vi "诊断标定3 - 副本.vi"(8 "CAN端口":u16(ring), 9 "设备索引号":u16(ring), 10 "CAN卡类型":u32(ring)=21) -> ()   [LabVIEW 2013] (continued)
                n2793 = local read "CAN卡类型"() -> (w3541:u32)
                n2794 = local read "CAN端口"() -> (w3539:u16)
                n2795 = call "标定授权发送.vi"("CAN卡类型"=w3541, "解锁类型"=enum16{"读取", "写", "下载"}."写", "设备索引号"=w3540, "CAN端口"=w3539, "是否连接"=TRUE, "板选择"=0, "FUNC"=w3543) -> ("发送成功"=w3546:bool)  [unwired: 8 out]
              }
              frame Enabled {
              }
            }
            n2796 = case shown="真" w3533 {
              tunnel: w3537 -> [w3551 w3556]
              tunnel: w3536 -> [w3550 w3555]
              tunnel: [w3551 w3553] -> w3535
              tunnel: [w3550 w3552] -> w3534
              frame False {
              }
              frame True {
                n2797 = Enqueue Element(queue=w3556, element="读取故障状态" ("元素"), error in (no error)=w3555) -> (queue out=w3553:refnum<queue>, error out=w3552:errorcluster)  [unwired: 2 out]
              }
            }
            n2798 = local write "电池故障"(string[][] []) -> ()
            n2799 = global write "EV05全局变量1.vi" "流控帧 2"(TRUE ("流控帧")) -> ()
            n2800 = local write "写?"(FALSE ("写?")) -> ()
            n2801 = local write "控制1"(TRUE ("控制1")) -> ()
            n2802 = local write "消除"(TRUE ("消除")) -> ()
            n2803 = local write "清BUFF"(FALSE ("清BUFF")) -> ()
            n2804 = global write "EV05全局变量1.vi" "流控帧"(FALSE ("流控帧")) -> ()
            n2805 = call <vilib>:"Set Busy.vi"("disable click? (T)"=FALSE) -> ()  [unwired: 3 in, 8 out]
          }
        }
      }
      event "项目软本读取": Value Change {
        n2806 = event-data() -> ("NewVal"=w3561:bool)  [unwired: 5 out]
        n2807 = case shown="真" w3561 {
          tunnel: w3560 -> [w3563 w3570]
          tunnel: w3559 -> [w3562 w3569]
          tunnel: [w3563 w3568] -> w3558
          tunnel: [w3562 w3567] -> w3557
          frame False {
          }
          frame True {
            n2808 = global read "EV05全局变量1.vi" "授权功能"() -> (w3565:bool)
            n2809 = case shown="假" w3565 {
              tunnel: [TRUE ("发送成功") w3589] -> w3566
              frame False {
              }
              frame True {
                n2810 = local read "设备索引号"() -> (w3584:u16)
                n2811 = local read "CAN卡类型"() -> (w3585:u32)
                n2812 = local read "CAN端口"() -> (w3583:u16)
                n2813 = call "标定授权发送.vi"("CAN卡类型"=w3585, "解锁类型"=enum16{"读取", "写", "下载"}."读取", "设备索引号"=w3584, "CAN端口"=w3583, "是否连接"=TRUE, "板选择"=0, "FUNC"=u32 0) -> ("发送成功"=w3589:bool)  [unwired: 8 out]
              }
            }
            n2814 = stacked-sequence {
              tunnel: [w3573] -> w3564
              frame #0 {
                w3573 = FALSE ("disable click? (T)")
                w3576 = FALSE ("写?")
                n2815 = local write "写?"(w3576) -> ()
                n2816 = global write "EV05全局变量1.vi" "写入超时"(w3576) -> ()
                n2817 = local write "项目软件版本号"(" " ("项目软件版本号")) -> ()
                n2818 = global write "EV05全局变量1.vi" "流控帧"(FALSE ("流控帧")) -> ()
                n2819 = local write "主从选择"(enum32{"主板", "从板"}."主板" ("主从选择")) -> ()
                n2820 = call <vilib>:"Set Busy.vi"("disable click? (T)"=w3573) -> ()  [unwired: 3 in, 8 out]
                n2821 = local write "清BUFF"(FALSE ("清BUFF")) -> ()
                n2822 = property on="保存版本信息" class="Bool (严格)"("Visible"=TRUE ("可见")) -> ()  [unwired: 2 in, 2 out]
                n2823 = global write "EV05全局变量1.vi" "流控帧 2"(TRUE ("流控帧 2")) -> ()
                n2824 = local write "控制1"(TRUE ("控制1")) -> ()
                n2825 = local write "消除"(TRUE ("消除")) -> ()
              }
            }
            n2826 = case shown="真" w3566 {
              tunnel: w3570 -> [w3591 w3596]
              tunnel: w3569 -> [w3590 w3595]
              tunnel: [w3591 w3593] -> w3568
              tunnel: [w3590 w3592] -> w3567
              tunnel: w3564 -> [_ _]
              frame False {
              }
              frame True {
                n2827 = Enqueue Element(queue=w3596, element="项目软件版本读取" ("元素"), error in (no error)=w3595) -> (queue out=w3593:refnum<queue>, error out=w3592:errorcluster)  [unwired: 2 out]
              }
            }
          }
        }
      }
      event "读硬件版本号": Value Change {
        n2828 = event-data() -> ("NewVal"=w3601:bool)  [unwired: 5 out]
        n2829 = case shown="真" w3601 {
          tunnel: w3600 -> [w3603 w3610]
          tunnel: w3599 -> [w3602 w3609]
          tunnel: [w3603 w3608] -> w3598
          tunnel: [w3602 w3607] -> w3597
          frame False {
          }
          frame True {
            n2830 = global read "EV05全局变量1.vi" "授权功能"() -> (w3605:bool)
            n2831 = case shown="假" w3605 {
              tunnel: [TRUE ("发送成功") w3629] -> w3606
              frame False {
              }
              frame True {
                n2832 = local read "设备索引号"() -> (w3624:u16)
                n2833 = local read "CAN卡类型"() -> (w3625:u32)
                n2834 = local read "CAN端口"() -> (w3623:u16)
                n2835 = call "标定授权发送.vi"("CAN卡类型"=w3625, "解锁类型"=enum16{"读取", "写", "下载"}."读取", "设备索引号"=w3624, "CAN端口"=w3623, "是否连接"=TRUE, "板选择"=0, "FUNC"=u32 0) -> ("发送成功"=w3629:bool)  [unwired: 8 out]
              }
            }
            n2836 = stacked-sequence {
              tunnel: [w3613] -> w3604
              frame #0 {
                w3613 = TRUE ("控制1")
                w3617 = FALSE ("写?")
                n2837 = local write "写?"(w3617) -> ()
                n2838 = global write "EV05全局变量1.vi" "写入超时"(w3617) -> ()
                n2839 = call <vilib>:"Set Busy.vi"("disable click? (T)"=FALSE) -> ()  [unwired: 3 in, 8 out]
                n2840 = local write "硬件版本号"("" ("硬件版本号")) -> ()
                n2841 = property on="保存版本信息" class="Bool (严格)"("Visible"=TRUE ("可见")) -> ()  [unwired: 2 in, 2 out]
                n2842 = local write "主从选择"(enum32{"主板", "从板"}."主板" ("主从选择")) -> ()
                n2843 = local write "控制1"(w3613) -> ()
                n2844 = local write "清BUFF"(FALSE ("清BUFF")) -> ()
                n2845 = global write "EV05全局变量1.vi" "流控帧 2"(TRUE ("流控帧 2")) -> ()
                n2846 = local write "消除"(TRUE ("消除")) -> ()
                n2847 = global write "EV05全局变量1.vi" "流控帧"(FALSE ("流控帧")) -> ()
              }
            }
            n2848 = case shown="真" w3606 {
              tunnel: w3610 -> [w3631 w3636]
              tunnel: w3609 -> [w3630 w3635]
              tunnel: [w3631 w3633] -> w3608
              tunnel: [w3630 w3632] -> w3607
              tunnel: w3604 -> [_ _]
              frame False {
              }
              frame True {
                n2849 = Enqueue Element(queue=w3636, element="硬件版本读取" ("元素"), error in (no error)=w3635) -> (queue out=w3633:refnum<queue>, error out=w3632:errorcluster)  [unwired: 2 out]
              }
            }
          }
        }
      }
      event "平台软件版本读取": Value Change {
        n2850 = event-data() -> ("NewVal"=w3641:bool)  [unwired: 5 out]
        n2851 = case shown="真" w3641 {
          tunnel: w3640 -> [w3643 w3650]
          tunnel: w3639 -> [w3642 w3649]
          tunnel: [w3643 w3648] -> w3638
          tunnel: [w3642 w3647] -> w3637
          frame False {
          }
          frame True {
            n2852 = global read "EV05全局变量1.vi" "授权功能"() -> (w3645:bool)
            n2853 = case shown="假" w3645 {
              tunnel: [TRUE ("发送成功") w3669] -> w3646
              frame False {
              }
              frame True {
                n2854 = local read "设备索引号"() -> (w3664:u16)
                n2855 = local read "CAN卡类型"() -> (w3665:u32)
                n2856 = local read "CAN端口"() -> (w3663:u16)
                n2857 = call "标定授权发送.vi"("CAN卡类型"=w3665, "解锁类型"=enum16{"读取", "写", "下载"}."读取", "设备索引号"=w3664, "CAN端口"=w3663, "是否连接"=TRUE, "板选择"=0, "FUNC"=u32 0) -> ("发送成功"=w3669:bool)  [unwired: 8 out]
              }
            }
            n2858 = stacked-sequence {
              tunnel: [w3653] -> w3644
              frame #0 {
                w3653 = TRUE ("控制1")
                w3657 = FALSE ("写?")
                n2859 = call <vilib>:"Set Busy.vi"("disable click? (T)"=FALSE) -> ()  [unwired: 3 in, 8 out]
                n2860 = local write "写?"(w3657) -> ()
                n2861 = global write "EV05全局变量1.vi" "写入超时"(w3657) -> ()
                n2862 = local write "平台软件版本号"(" " ("平台软件版本号")) -> ()
                n2863 = local write "控制1"(w3653) -> ()
                n2864 = local write "消除"(TRUE ("消除")) -> ()
                n2865 = property on="保存版本信息" class="Bool (严格)"("Visible"=TRUE ("可见")) -> ()  [unwired: 2 in, 2 out]
                n2866 = global write "EV05全局变量1.vi" "流控帧 2"(TRUE ("流控帧 2")) -> ()
                n2867 = local write "主从选择"(enum32{"主板", "从板"}."主板" ("主从选择")) -> ()
                n2868 = local write "清BUFF"(FALSE ("清BUFF")) -> ()
                n2869 = global write "EV05全局变量1.vi" "流控帧"(FALSE ("流控帧")) -> ()
              }
            }
            n2870 = case shown="真" w3646 {
              tunnel: w3650 -> [w3671 w3676]
              tunnel: w3649 -> [w3670 w3675]
              tunnel: [w3671 w3673] -> w3648
              tunnel: [w3670 w3672] -> w3647
              tunnel: w3644 -> [_ _]
              frame False {
              }
              frame True {
                n2871 = Enqueue Element(queue=w3676, element="平台软件版本读取" ("元素"), error in (no error)=w3675) -> (queue out=w3673:refnum<queue>, error out=w3672:errorcluster)  [unwired: 2 out]
              }
            }
          }
        }
      }
      event "模块版本读取": Value Change {
        n2872 = event-data() -> ("NewVal"=w3681:bool)  [unwired: 5 out]
        n2873 = case shown="真" w3681 {
          tunnel: w3680 -> [w3683 w3690]
          tunnel: w3679 -> [w3682 w3689]
          tunnel: [w3683 w3688] -> w3678
          tunnel: [w3682 w3687] -> w3677
          frame False {
          }
          frame True {
            n2874 = global read "EV05全局变量1.vi" "授权功能"() -> (w3685:bool)
            n2875 = case shown="假" w3685 {
              tunnel: [TRUE ("发送成功") w3708] -> w3686
              frame False {
              }
              frame True {
                n2876 = local read "设备索引号"() -> (w3703:u16)
                n2877 = local read "CAN卡类型"() -> (w3704:u32)
                n2878 = local read "CAN端口"() -> (w3702:u16)
                n2879 = call "标定授权发送.vi"("CAN卡类型"=w3704, "解锁类型"=enum16{"读取", "写", "下载"}."读取", "设备索引号"=w3703, "CAN端口"=w3702, "是否连接"=TRUE, "板选择"=0, "FUNC"=u32 0) -> ("发送成功"=w3708:bool)  [unwired: 8 out]
              }
            }
            n2880 = stacked-sequence {
              tunnel: [w3693] -> w3684
              frame #0 {
                w3693 = TRUE ("控制1")
                w3696 = FALSE ("写?")
                n2881 = call <vilib>:"Set Busy.vi"("disable click? (T)"=FALSE) -> ()  [unwired: 3 in, 8 out]
                n2882 = local write "写?"(w3696) -> ()
                n2883 = global write "EV05全局变量1.vi" "写入超时"(w3696) -> ()
                n2884 = local write "主从选择"(enum32{"主板", "从板"}."主板" ("主从选择")) -> ()
                n2885 = local write "清BUFF"(FALSE ("清BUFF")) -> ()
                n2886 = property on="保存版本信息" class="Bool (严格)"("Visible"=TRUE ("可见")) -> ()  [unwired: 2 in, 2 out]
                n2887 = global write "EV05全局变量1.vi" "流控帧 2"(TRUE ("流控帧 2")) -> ()
                n2888 = local write "控制1"(w3693) -> ()
                n2889 = local write "消除"(TRUE ("消除")) -> ()
                n2890 = global write "EV05全局变量1.vi" "流控帧"(FALSE ("流控帧")) -> ()
              }
            }
            n2891 = case shown="真" w3686 {
              tunnel: w3690 -> [w3710 w3715]
              tunnel: w3689 -> [w3709 w3714]
              tunnel: [w3710 w3712] -> w3688
              tunnel: [w3709 w3711] -> w3687
              tunnel: w3684 -> [_ _]
              frame False {
              }
              frame True {
                n2892 = Enqueue Element(queue=w3715, element="模块软件版本读取" ("元素"), error in (no error)=w3714) -> (queue out=w3712:refnum<queue>, error out=w3711:errorcluster)  [unwired: 2 out]
              }
            }
          }
        }
      }
      event "保存版本信息": Value Change {
        n2893 = event-data() -> ("NewVal"=w3716:bool)  [unwired: 6 out]
        n2894 = case shown="真" w3716 {
          frame False {
          }
          frame True {
            n2895 = stacked-sequence {
              seq-local: [w3720 _] -> [_ w3722]
              seq-local: [w3719 _] -> [_ w3721]
              frame #0 {
                n2896 = call "请输入从板个数"() -> ("从板个数"=w3720:dbl, "确定"=w3719:bool)  [unwired: 17 in, 1 out]
              }
              frame #1 {
                n2897 = case shown="真" w3721 {
                  tunnel: w3722 -> [_ w3725]
                  frame False {
                  }
                  frame True {
                    n2898 = call <vilib>:"Application Directory.vi"() -> ("Application Directory"=w3737:path)
                    n2899 = Build Path(base path=w3737, name or relative path="SaveData" ("名称或相对路径")) -> (appended path=w3735:path)
                    n2900 = local read "模块版本名称"() -> (w3730:string[][])
                    n2901 = local read "项目软件版本"() -> (w3727:string[])
                    n2902 = local read "模块版本值"() -> (w3729:string[][])
                    n2903 = local read "平台软件版本"() -> (w3726:string[])
                    n2904 = local read "模块个数"() -> (w3723:u8[])
                    n2905 = local read "硬件版本"() -> (w3728:string[])
                    n2906 = call "文件对话框3"("start path"=w3735, "prompt"="选择要保存数据的位置", "default name"="BMS版本信息.txt") -> ("selected path"=w3731:path, "cancelled"=w3732:bool)  [unwired: 9 in, 2 out]
                    n2907 = Increment(x=w3725) -> (x+1=w3724:dbl)
                    n2908 = for {
                      N: w3724 -> [_]
                      tunnel: w3732 -> [w3753]
                      tunnel: w3731 -> [w3752]
                      tunnel: w3730 -> [w3742] mode=indexing
                      tunnel: w3729 -> [w3740] mode=indexing
                      tunnel: w3728 -> [w3747] mode=indexing
                      tunnel: w3727 -> [w3746] mode=indexing
                      tunnel: w3726 -> [w3745] mode=indexing
                      tunnel: w3723 -> [w3738] mode=indexing
                      i -> [w3744]
                      w3750 = ""
                      w3757 = 0 ("索引")
                      n2909 = case shown="0, 默认" w3744 {
                        selector: w3744 -> [_ w3771]
                        tunnel: ["主板版本信息" w3772] -> w3762
                        tunnel: [FALSE TRUE] -> w3748
                        frame 0, Default {
                        }
                        frame 1.. {
                          n2910 = Number To Decimal String(number=w3771) -> (decimal integer string=w3770:string)  [unwired: 1 in]
                          n2911 = Concatenate Strings("从板", w3770, "版本信息") -> (w3772:string)
                        }
                      }
                      n2912 = Increment(x=w3738) -> (x+1=w3739:u8)
                      n2913 = Array Subset(array=w3742, length=w3739) -> (w3743:string[])  [unwired: 1 in]
                      n2914 = Array Subset(array=w3740, length=w3739) -> (w3741:string[])  [unwired: 1 in]
                      n2915 = Build Array(w3750, w3745, w3746, w3747, w3750) -> (w3756:string[])
                      n2916 = Build Array(w3762, "平台软件版本号", "项目软件版本号", "硬件版本号", "模块版本号") -> (w3758:string[])
                      n2917 = Insert Into Array(array=w3743, index=w3757, new element=w3758) -> (w3755:string[])
                      n2918 = Insert Into Array(array=w3741, index=w3757, new element=w3756) -> (w3754:string[])
                      n2919 = Build Array(w3755, w3754) -> (w3751:string[][])
                      n2920 = case shown="假" w3753 {
                        tunnel: w3752 -> [w3766 _]
                        tunnel: w3751 -> [w3765 _]
                        tunnel: w3748 -> [w3763 _]
                        frame False {
                          n2921 = call-poly <vilib>:"Write To Spreadsheet File.vi"("transpose? (no:F)"=TRUE, "append to file? (new file:F)"=w3763, "2D data"=w3765, "file path (dialog if empty)"=w3766) -> ()  [unwired: 4 in, 1 out]
                        }
                        frame True {
                        }
                      }
                    }
                  }
                }
              }
            }
          }
        }
      }
      event "单个写入": Value Change {
        n2922 = event-data() -> ("NewVal"=w3779:bool)  [unwired: 5 out]
        n2923 = case shown="真" w3779 {
          tunnel: w3778 -> [w3781 w3788]
          tunnel: w3777 -> [w3780 w3787]
          tunnel: [w3781 w3786] -> w3776
          tunnel: [w3780 w3785] -> w3775
          frame False {
          }
          frame True {
            w3783 = FALSE ("流控帧")
            w3782 = TRUE ("流控帧 2")
            n2924 = disable-structure shown="禁用" {
              disable-tunnel: [w3797 TRUE ("发送成功")] -> w3784
              frame Disabled {
                n2925 = local read "主从选择"() -> (w3789:enum32{"主板", "从板"})
                n2926 = case shown="\"主板\", 默认" w3789 {
                  tunnel: [0.0 ("FUNC") w3799] -> w3794
                  frame "主板", Default {
                  }
                  frame "从板" {
                    n2927 = local read "从板号"() -> (w3799:u8)
                  }
                }
                n2928 = local read "设备索引号"() -> (w3791:u16)
                n2929 = local read "CAN卡类型"() -> (w3792:u32)
                n2930 = local read "CAN端口"() -> (w3790:u16)
                n2931 = call "标定授权发送.vi"("CAN卡类型"=w3792, "解锁类型"=enum16{"读取", "写", "下载"}."写", "设备索引号"=w3791, "CAN端口"=w3790, "是否连接"=TRUE, "板选择"=0, "FUNC"=w3794) -> ("发送成功"=w3797:bool)  [unwired: 8 out]
              }
              frame Enabled {
              }
            }
            n2932 = case shown="真" w3784 {
              tunnel: w3788 -> [w3802 w3806]
              tunnel: w3787 -> [w3801 w3805]
              tunnel: [w3802 w3808] -> w3786
              tunnel: [w3801 w3807] -> w3785
              frame False {
              }
              frame True {
                n2933 = Flush Queue(queue=w3806, error in (no error)=w3805) -> (queue out=w3804:refnum<queue>, error out=w3803:errorcluster)  [unwired: 1 out]
                n2934 = Enqueue Element(queue=w3804, element="单个写入" ("元素"), error in (no error)=w3803) -> (queue out=w3808:refnum<queue>, error out=w3807:errorcluster)  [unwired: 2 out]
              }
            }
            n2935 = global write "EV05全局变量1.vi" "读取超时"(w3783) -> ()
            n2936 = global write "EV05全局变量1.vi" "流控帧"(w3783) -> ()
            n2937 = local write "消除"(w3782) -> ()
            n2938 = local write "控制1"(w3782) -> ()
            n2939 = global write "EV05全局变量1.vi" "流控帧 2"(w3782) -> ()
            n2940 = local write "写?"(w3782) -> ()
          }
        }
      }
      event "全部写入": Value Change {
        n2941 = event-data() -> ("NewVal"=w3814:bool)  [unwired: 5 out]
        n2942 = case shown="真" w3814 {
          tunnel: w3813 -> [w3816 w3824]
          tunnel: w3812 -> [w3815 w3823]
          tunnel: [w3816 w3822] -> w3811
          tunnel: [w3815 w3821] -> w3810
          frame False {
          }
          frame True {
            w3818 = FALSE ("流控帧")
            w3817 = TRUE ("流控帧 2")
            n2943 = global read "EV05全局变量1.vi" "授权功能"() -> (w3819:bool)
            n2944 = case shown="真" w3819 {
              tunnel: [TRUE ("发送成功") w3834] -> w3820
              frame False {
              }
              frame True {
                n2945 = local read "主从选择"() -> (w3826:enum32{"主板", "从板"})
                n2946 = case shown="\"从板\"" w3826 {
                  tunnel: [0.0 ("FUNC") w3836] -> w3827
                  frame "主板", Default {
                  }
                  frame "从板" {
                    n2947 = local read "从板号"() -> (w3836:u8)
                  }
                }
                n2948 = local read "设备索引号"() -> (w3829:u16)
                n2949 = local read "CAN卡类型"() -> (w3830:u32)
                n2950 = local read "CAN端口"() -> (w3828:u16)
                n2951 = call "标定授权发送.vi"("CAN卡类型"=w3830, "解锁类型"=enum16{"读取", "写", "下载"}."写", "设备索引号"=w3829, "CAN端口"=w3828, "是否连接"=TRUE, "板选择"=0, "FUNC"=w3827) -> ("发送成功"=w3834:bool)  [unwired: 8 out]
              }
            }
            n2952 = case shown="真" w3820 {
              tunnel: w3824 -> [w3838 w3842]
              tunnel: w3823 -> [w3837 w3841]
              tunnel: [w3838 w3844] -> w3822
              tunnel: [w3837 w3843] -> w3821
              frame False {
              }
              frame True {
                n2953 = Flush Queue(queue=w3842, error in (no error)=w3841) -> (queue out=w3840:refnum<queue>, error out=w3839:errorcluster)  [unwired: 1 out]
                n2954 = Enqueue Element(queue=w3840, element="全部写入" ("元素"), error in (no error)=w3839) -> (queue out=w3844:refnum<queue>, error out=w3843:errorcluster)  [unwired: 1 in, 1 out]
              }
            }
            n2955 = global write "EV05全局变量1.vi" "读取超时"(w3818) -> ()
            n2956 = global write "EV05全局变量1.vi" "流控帧"(w3818) -> ()
            n2957 = local write "消除"(w3817) -> ()
            n2958 = local write "控制1"(w3817) -> ()
            n2959 = global write "EV05全局变量1.vi" "流控帧 2"(w3817) -> ()
            n2960 = local write "写?"(w3817) -> ()
          }
        }
      }
      event "单个读取": Value Change {
        n2961 = event-data() -> ("NewVal"=w3850:bool)  [unwired: 5 out]
        n2962 = case shown="真" w3850 {
          tunnel: w3849 -> [w3852 w3860]
          tunnel: w3848 -> [w3851 w3859]
          tunnel: [w3852 w3858] -> w3847
          tunnel: [w3851 w3857] -> w3846
          frame False {
          }
          frame True {
            w3853 = FALSE ("流控帧")
            w3854 = TRUE ("流控帧 2")
            n2963 = global read "EV05全局变量1.vi" "授权功能"() -> (w3855:bool)
            n2964 = case shown="假" w3855 {
              tunnel: [TRUE ("发送成功") w3869] -> w3856
              frame False {
              }
              frame True {
                n2965 = local read "设备索引号"() -> (w3863:u16)
                n2966 = local read "CAN卡类型"() -> (w3864:u32)
                n2967 = local read "CAN端口"() -> (w3862:u16)
                n2968 = call "标定授权发送.vi"("CAN卡类型"=w3864, "解锁类型"=enum16{"读取", "写", "下载"}."读取", "设备索引号"=w3863, "CAN端口"=w3862, "是否连接"=TRUE, "板选择"=0, "FUNC"=u32 1) -> ("发送成功"=w3869:bool)  [unwired: 8 out]
              }
            }
            n2969 = case shown="真" w3856 {
              tunnel: w3860 -> [w3871 w3875]
              tunnel: w3859 -> [w3870 w3873]
              tunnel: [w3871 w3877] -> w3858
              tunnel: [w3870 w3876] -> w3857
              frame False {
              }
              frame True {
                n2970 = Flush Queue(queue=w3875, error in (no error)=w3873) -> (queue out=w3874:refnum<queue>, error out=w3872:errorcluster)  [unwired: 1 out]
                n2971 = Enqueue Element(queue=w3874, element="单个读取" ("元素"), error in (no error)=w3872) -> (queue out=w3877:refnum<queue>, error out=w3876:errorcluster)  [unwired: 2 out]
              }
            }
            n2972 = global write "EV05全局变量1.vi" "写入超时"(w3853) -> ()
            n2973 = global write "EV05全局变量1.vi" "流控帧"(w3853) -> ()
            n2974 = local write "写?"(w3853) -> ()
            n2975 = local write "消除"(w3854) -> ()
            n2976 = local write "控制1"(w3854) -> ()
            n2977 = global write "EV05全局变量1.vi" "流控帧 2"(w3854) -> ()
          }
        }
      }
      event "全部读取": Value Change {
        n2978 = event-data() -> ("NewVal"=w3883:bool)  [unwired: 5 out]
        n2979 = case shown="真" w3883 {
          tunnel: w3882 -> [w3885 w3889]
          tunnel: w3881 -> [w3884 w3888]
          tunnel: [w3885 w3887] -> w3880
          tunnel: [w3884 w3886] -> w3879
          frame False {
          }
          frame True {
            n2980 = stacked-sequence {
              seq-local: [w3894 _] -> [_ _]
              seq-local: [w3893 _] -> [_ _]
              tunnel: w3889 -> [w3896 w3926]
              tunnel: w3888 -> [w3895 w3925]
              tunnel: [_ w3930] -> w3887
              tunnel: [_ w3929] -> w3886
              frame #0 {
                w3890 = FALSE ("布尔")
                n2981 = local read "路径"() -> (w3892:path)
                n2982 = Empty String/Path?(string/path=w3892) -> (empty?=w3891:bool)
                n2983 = case shown="假" w3891 {
                  tunnel: w3896 -> [w3904 w3922]
                  tunnel: w3895 -> [w3903 w3921]
                  tunnel: [w3900 w3921] -> w3894
                  tunnel: [w3899 w3922] -> w3893
                  frame False {
                    n2984 = global read "EV05全局变量1.vi" "授权功能"() -> (w3901:bool)
                    n2985 = case shown="真" w3901 {
                      tunnel: [TRUE ("发送成功") w3913] -> w3902
                      frame False {
                      }
                      frame True {
                        n2986 = local read "设备索引号"() -> (w3907:u16)
                        n2987 = local read "CAN卡类型"() -> (w3908:u32)
                        n2988 = local read "CAN端口"() -> (w3906:u16)
                        n2989 = call "标定授权发送.vi"("CAN卡类型"=w3908, "解锁类型"=enum16{"读取", "写", "下载"}."读取", "设备索引号"=w3907, "CAN端口"=w3906, "是否连接"=TRUE, "板选择"=0, "FUNC"=u32 1) -> ("发送成功"=w3913:bool)  [unwired: 8 out]
                      }
                    }
                    n2990 = case shown="真" w3902 {
                      tunnel: w3904 -> [w3915 w3920]
                      tunnel: w3903 -> [w3914 w3919]
                      tunnel: [w3915 w3917] -> w3899
                      tunnel: [w3914 w3916] -> w3900
                      frame False {
                      }
                      frame True {
                        n2991 = Enqueue Element(queue=w3920, element="读配置文件" ("元素"), error in (no error)=w3919) -> (queue out=w3917:refnum<queue>, error out=w3916:errorcluster)  [unwired: 2 out]
                      }
                    }
                    n2992 = local write "布尔"(FALSE ("布尔")) -> ()
                    n2993 = Wait Until Next ms Multiple(millisecond multiple=u32 200 ("毫秒倍数")) -> ()  [unwired: 1 out]
                  }
                  frame True {
                  }
                }
                n2994 = local write "1 6"(w3890) -> ()
                n2995 = local write "1 7"(w3890) -> ()
                n2996 = local write "1 8"(w3890) -> ()
                n2997 = local write "1 9"(w3890) -> ()
                n2998 = local write "1 10"(w3890) -> ()
                n2999 = local write "1 12"(w3890) -> ()
              }
              frame #1 {
                w3923 = FALSE ("流控帧")
                w3924 = TRUE ("流控帧 2")
                n3000 = global read "EV05全局变量1.vi" "授权功能"() -> (w3927:bool)
                n3001 = case shown="假" w3927 {
                  tunnel: [TRUE ("发送成功") w3939] -> w3928
                  frame False {
                  }
                  frame True {
                    n3002 = local read "设备索引号"() -> (w3933:u16)
                    n3003 = local read "CAN卡类型"() -> (w3934:u32)
                    n3004 = local read "CAN端口"() -> (w3932:u16)
                    n3005 = call "标定授权发送.vi"("CAN卡类型"=w3934, "解锁类型"=enum16{"读取", "写", "下载"}."读取", "设备索引号"=w3933, "CAN端口"=w3932, "是否连接"=TRUE, "板选择"=0, "FUNC"=u32 1) -> ("发送成功"=w3939:bool)  [unwired: 8 out]
                  }
                }
                n3006 = case shown="真" w3928 {
                  tunnel: w3926 -> [w3941 w3942]
                  tunnel: w3925 -> [w3940 w3945]
                  tunnel: [w3941 w3947] -> w3930
                  tunnel: [w3940 w3946] -> w3929
                  frame False {
                  }
                  frame True {
                    n3007 = Flush Queue(queue=w3942, error in (no error)=w3945) -> (queue out=w3943:refnum<queue>, error out=w3944:errorcluster)  [unwired: 1 out]
                    n3008 = Enqueue Element(queue=w3943, element="全部读取" ("元素"), error in (no error)=w3944) -> (queue out=w3947:refnum<queue>, error out=w3946:errorcluster)  [unwired: 2 out]
                  }
                }
                n3009 = global write "EV05全局变量1.vi" "写入超时"(w3923) -> ()
                n3010 = global write "EV05全局变量1.vi" "流控帧"(w3923) -> ()
                n3011 = local write "写?"(w3923) -> ()
                n3012 = local write "消除"(w3924) -> ()
                n3013 = local write "控制1"(w3924) -> ()
                n3014 = global write "EV05全局变量1.vi" "流控帧 2"(w3924) -> ()
              }
            }
          }
        }
      }
      event "开启均衡": Value Change {
        n3015 = event-data() -> ("NewVal"=w3953:bool)  [unwired: 5 out]
        n3016 = case shown="真" w3953 {
          tunnel: w3952 -> [w3955 w3962]
          tunnel: w3951 -> [w3954 w3961]
          tunnel: [w3955 w3960] -> w3950
          tunnel: [w3954 w3959] -> w3949
          frame False {
          }
          frame True {
            n3017 = global read "EV05全局变量1.vi" "授权功能"() -> (w3957:bool)
            n3018 = case shown="假" w3957 {
              tunnel: [TRUE ("发送成功") w3972] -> w3958
              frame False {
              }
              frame True {
                n3019 = local read "主从选择"() -> (w3964:enum32{"主板", "从板"})
                n3020 = case shown="\"从板\"" w3964 {
                  tunnel: [0.0 ("FUNC") w3974] -> w3965
                  frame "主板", Default {
                  }
                  frame "从板" {
                    n3021 = local read "从板号"() -> (w3974:u8)
                  }
                }
                n3022 = local read "设备索引号"() -> (w3967:u16)
                n3023 = local read "CAN卡类型"() -> (w3968:u32)
                n3024 = local read "CAN端口"() -> (w3966:u16)
                n3025 = call "标定授权发送.vi"("CAN卡类型"=w3968, "解锁类型"=enum16{"读取", "写", "下载"}."写", "设备索引号"=w3967, "CAN端口"=w3966, "是否连接"=TRUE, "板选择"=0, "FUNC"=w3965) -> ("发送成功"=w3972:bool)  [unwired: 8 out]
              }
            }
            n3026 = case shown="真" w3958 {
              tunnel: w3962 -> [w3976 w3981]
              tunnel: w3961 -> [w3975 w3980]
              tunnel: [w3976 w3978] -> w3960
              tunnel: [w3975 w3977] -> w3959
              frame False {
              }
              frame True {
                n3027 = Enqueue Element(queue=w3981, element="开启均衡" ("元素"), error in (no error)=w3980) -> (queue out=w3978:refnum<queue>, error out=w3977:errorcluster)  [unwired: 2 out]
              }
            }
            n3028 = call <vilib>:"Set Busy.vi"("disable click? (T)"=TRUE) -> ()  [unwired: 3 in, 8 out]
          }
        }
      }
      event "关闭均衡": Value Change {
        n3029 = event-data() -> ("NewVal"=w3986:bool)  [unwired: 5 out]
        n3030 = case shown="真" w3986 {
          tunnel: w3985 -> [w3988 w3995]
          tunnel: w3984 -> [w3987 w3994]
          tunnel: [w3988 w3993] -> w3983
          tunnel: [w3987 w3992] -> w3982
          frame False {
          }
          frame True {
            n3031 = global read "EV05全局变量1.vi" "授权功能"() -> (w3990:bool)
            n3032 = case shown="假" w3990 {
              tunnel: [TRUE ("发送成功") w4005] -> w3991
              frame False {
              }
              frame True {
                n3033 = local read "主从选择"() -> (w3997:enum32{"主板", "从板"})
                n3034 = case shown="\"从板\"" w3997 {
                  tunnel: [0.0 ("FUNC") w4007] -> w3998
                  frame "主板", Default {
                  }
                  frame "从板" {
                    n3035 = local read "从板号"() -> (w4007:u8)
                  }
                }
                n3036 = local read "设备索引号"() -> (w4000:u16)
                n3037 = local read "CAN卡类型"() -> (w4001:u32)
                n3038 = local read "CAN端口"() -> (w3999:u16)
                n3039 = call "标定授权发送.vi"("CAN卡类型"=w4001, "解锁类型"=enum16{"读取", "写", "下载"}."写", "设备索引号"=w4000, "CAN端口"=w3999, "是否连接"=TRUE, "板选择"=0, "FUNC"=w3998) -> ("发送成功"=w4005:bool)  [unwired: 8 out]
              }
            }
            n3040 = case shown="真" w3991 {
              tunnel: w3995 -> [w4009 w4014]
              tunnel: w3994 -> [w4008 w4013]
              tunnel: [w4009 w4011] -> w3993
              tunnel: [w4008 w4010] -> w3992
              frame False {
              }
              frame True {
                n3041 = Enqueue Element(queue=w4014, element="关闭均衡" ("元素"), error in (no error)=w4013) -> (queue out=w4011:refnum<queue>, error out=w4010:errorcluster)  [unwired: 2 out]
              }
            }
            n3042 = call <vilib>:"Set Busy.vi"("disable click? (T)"=TRUE) -> ()  [unwired: 3 in, 8 out]
          }
        }
      }
      event "强制开启均衡": Value Change {
        n3043 = event-data() -> ("NewVal"=w4019:bool)  [unwired: 5 out]
        n3044 = case shown="真" w4019 {
          tunnel: w4018 -> [w4021 w4028]
          tunnel: w4017 -> [w4020 w4027]
          tunnel: [w4021 w4026] -> w4016
          tunnel: [w4020 w4025] -> w4015
          frame False {
          }
          frame True {
            n3045 = global read "EV05全局变量1.vi" "授权功能"() -> (w4023:bool)
            n3046 = case shown="假" w4023 {
              tunnel: [TRUE ("发送成功") w4038] -> w4024
              frame False {
              }
              frame True {
                n3047 = local read "主从选择"() -> (w4030:enum32{"主板", "从板"})
                n3048 = case shown="\"从板\"" w4030 {
                  tunnel: [0.0 ("FUNC") w4040] -> w4031
                  frame "主板", Default {
                  }
                  frame "从板" {
                    n3049 = local read "从板号"() -> (w4040:u8)
                  }
                }
                n3050 = local read "设备索引号"() -> (w4033:u16)
                n3051 = local read "CAN卡类型"() -> (w4034:u32)
                n3052 = local read "CAN端口"() -> (w4032:u16)
                n3053 = call "标定授权发送.vi"("CAN卡类型"=w4034, "解锁类型"=enum16{"读取", "写", "下载"}."写", "设备索引号"=w4033, "CAN端口"=w4032, "是否连接"=TRUE, "板选择"=0, "FUNC"=w4031) -> ("发送成功"=w4038:bool)  [unwired: 8 out]
              }
            }
            n3054 = case shown="真" w4024 {
              tunnel: w4028 -> [w4042 w4047]
              tunnel: w4027 -> [w4041 w4046]
              tunnel: [w4042 w4044] -> w4026
              tunnel: [w4041 w4043] -> w4025
              frame False {
              }
              frame True {
                n3055 = Enqueue Element(queue=w4047, element="强制均衡" ("元素"), error in (no error)=w4046) -> (queue out=w4044:refnum<queue>, error out=w4043:errorcluster)  [unwired: 2 out]
              }
            }
            n3056 = call <vilib>:"Set Busy.vi"("disable click? (T)"=TRUE) -> ()  [unwired: 3 in, 8 out]
          }
        }
      }
    }
    n3057 = Unbundle By Name(w1234) -> ("status"=w1233:bool)
    n3058 = Or(x=w1233, y=w1235) -> (x .or. y?=w1236:bool)
  }
  n3059 = while {
    tunnel: w36 -> [w4053]
    tunnel: w35 -> [w4052]
    stop <- w4049 stop-if-true
    n3060 = local read "停止"() -> (w4049:bool)
    n3061 = Dequeue Element(queue=w4053, timeout in ms (-1)=100 ("超时毫秒(-1)"), error in (no error)=w4052) -> (element=w4051:string, error out=w4050:errorcluster)  [unwired: 2 out]
    n3062 = case shown="无错误" w4050 {
      tunnel: w4051 -> [w4054 _]
      frame No Error {
        n3063 = case shown="\"单个读取\"" w4054 {
          frame "假", Default {
            n3064 = local write "强制终止读写标记"(FALSE ("强制终止读写标记")) -> ()
          }
          frame "单个写入" {
            n3065 = local read "主从选择"() -> (w4064:enum32{"主板", "从板"})
            n3066 = case shown="\"主板\", 默认" w4064 {
              tunnel: [w4075 w4090] -> w4061
              tunnel: [0.0 w4088] -> w4065
              tunnel: [_ w4089] -> w4063
              tunnel: [w4073 _] -> w4062
              frame "主板", Default {
                n3067 = flat-sequence {
                  tunnel: [w4087] -> w4073
                  frame #0 {
                    n3068 = control-ref of="高压参数"() -> (w4078:refnum<vi>)
                    n3069 = control-ref of="电池信息"() -> (w4079:refnum<vi>)
                    n3070 = control-ref of="一级故障"() -> (w4085:refnum<vi>)
                    n3071 = control-ref of="一级故障 2"() -> (w4083:refnum<vi>)
                    n3072 = control-ref of="一级故障 3"() -> (w4082:refnum<vi>)
                    n3073 = control-ref of="加热控制参数"() -> (w4081:refnum<vi>)
                    n3074 = control-ref of="充电控制参数"() -> (w4080:refnum<vi>)
                    n3075 = control-ref of="项目信息"() -> (w4084:refnum<vi>)
                    n3076 = control-ref of="项目信息2"() -> (w4086:refnum<vi>)
                    n3077 = local read "主板数据"() -> (w4076:T4)
                    n3078 = Bundle(cluster=w4076, "项目信息"=w4084, "一级故障 4"=w4086, "一级故障"=w4085, "一级故障 2"=w4083, "一级故障 3"=w4082, "加热控制参数"=w4081, "充电控制参数"=w4080, "高压参数"=w4078, "电池信息"=w4079) -> (w4077:T4)
                    n3079 = local write "主板数据"(w4077) -> ()
                  }
                  frame #1 {
                    n3080 = control-ref of="主板数据"() -> (w4087:refnum<vi>)
                  }
                }
                n3081 = local read "主板选项"() -> (w4075:string)
              }
              frame "从板" {
                n3082 = stacked-sequence {
                  tunnel: [_ w4101] -> w4089
                  frame #0 {
                    n3083 = control-ref of="从板号"() -> (w4100:refnum<vi>)
                    n3084 = control-ref of="项目信息 2"() -> (w4099:refnum<vi>)
                    n3085 = control-ref of="均衡参数"() -> (w4094:refnum<vi>)
                    n3086 = control-ref of="加热控制参数"() -> (w4098:refnum<vi>)
                    n3087 = control-ref of="一级故障(从板)"() -> (w4097:refnum<vi>)
                    n3088 = control-ref of="二级故障(从板)"() -> (w4096:refnum<vi>)
                    n3089 = control-ref of="三级故障(从板)"() -> (w4095:refnum<vi>)
                    n3090 = control-ref of="电池组信息"() -> (w4091:refnum<vi>)
                    n3091 = local read "从板信息"() -> (w4092:T2)
                    n3092 = Bundle(cluster=w4092, "从板号"=w4100, "项目信息 2"=w4099, "加热控制参数"=w4098, "一级故障(从板)"=w4097, "二级故障(从板)"=w4096, "三级故障(从板)"=w4095, "电池组信息(从板)"=w4091, "均衡参数"=w4094) -> (w4093:T2)
                    n3093 = local write "从板信息"(w4093) -> ()
                  }
                  frame #1 {
                    n3094 = control-ref of="从板信息"() -> (w4101:refnum<vi>)
                  }
                }
                n3095 = local read "从板选项"() -> (w4090:string)
                n3096 = local read "从板号"() -> (w4088:u8)
              }
            }
            n3097 = local read "从板个数"() -> (w4066:dbl)
            n3098 = local read "二维码信息 2"() -> (w4056:string)
            n3099 = local read "二维码信息"() -> (w4057:string)
            n3100 = local read "快换"() -> (w4067:bool)
            n3101 = call "输入数据解析.vi"("单个参数补充"=w4066, "从板号"=w4065, "主板二维码"=w4057, "从板二维码"=w4056, "主板引用"=w4062, "从板引用"=w4063, "主板选项"=w4061, "枚举"=w4064, "快换"=w4067) -> ("输出数组"=w4071:dbl[][], "数组长度"=w4070:dbl[], "循环次数"=w4060:i32, "命令"=w4069:u32, "名称"=w4059:string[], "命令序号"=w4068:u32[])  [unwired: 1 out]
            n3102 = for {
              N: w4060 -> [w4107]
              tunnel: w4071 -> [w4117]
              tunnel: w4070 -> [w4116]
              tunnel: w4069 -> [w4115]
              tunnel: w4068 -> [w4114]
              tunnel: w4065 -> [w4105]
              tunnel: w4061 -> [w4113]
              tunnel: w4059 -> [w4109]
              tunnel: [w4102] -> w4058
              i -> [w4108]
              n3103 = Index Array(array=w4117, index (row)=w4108) -> (element=w4112:dbl[])  [unwired: 1 in]
              n3104 = Index Array(array=w4116, index=w4108) -> (element=w4111:dbl)
              n3105 = Index Array(array=w4109, index=w4108) -> (element=w4106:string)
              n3106 = case shown="\"假\", 默认" w4106 {
                tunnel: [w4119 w4120] -> w4104
                tunnel: w4105 -> [w4119 _]
                tunnel: [TRUE ("确定") w4121] -> w4103
                frame "假", Default {
                }
                frame "从板号" {
                  n3107 = call "请输入当前从板板号"() -> ("当前从板板号"=w4120:dbl, "确定"=w4121:bool)  [unwired: 17 in, 1 out]
                  n3108 = local write "当前从板板号"(w4120) -> ()
                }
              }
              n3109 = Index Array(array=w4114, index=w4108) -> (element=w4110:u32)
              n3110 = global write "全局 1.vi" "名称"(w4106) -> ()
              n3111 = case shown="真" w4103 {
                tunnel: w4115 -> [_ w4131]
                tunnel: w4113 -> [_ w4130]
                tunnel: w4112 -> [_ w4129]
                tunnel: w4111 -> [_ w4128]
                tunnel: w4110 -> [_ w4127]
                tunnel: w4108 -> [_ w4126]
                tunnel: w4106 -> [_ w4125]
                tunnel: w4107 -> [_ w4124]
                tunnel: w4104 -> [_ w4123]
                tunnel: [_ w4122] -> w4102
                frame False {
                  n3112 = call <vilib>:"Unset Busy.vi"() -> ()  [unwired: 11 in, 1 out]
                }
                frame True {
                  n3113 = stacked-sequence {
                    seq-local: [_ _ _ w4159 _ _] -> [_ _ _ _ w4168 _]
                    tunnel: w4129 -> [_ _ w4144 _ _ _]
                    tunnel: w4128 -> [_ _ w4143 _ _ _]
                    tunnel: w4131 -> [_ _ w4137 _ _ _]
                    tunnel: w4127 -> [_ _ w4135 _ _ _]
                    tunnel: w4130 -> [_ _ _ _ _ _]
                    tunnel: w4126 -> [_ _ _ _ _ w4179]
                    tunnel: w4125 -> [_ _ _ _ w4167 _]
                    tunnel: w4124 -> [_ _ _ _ _ w4180]
                    tunnel: w4123 -> [_ _ w4136 _ _ _]
                    tunnel: [_ _ _ _ _ w4177] -> w4122
                    frame #0 {
                      w4133 = FALSE ("流控帧")
                      w4132 = TRUE ("流控帧 2")
                      n3114 = call <vilib>:"Set Busy.vi"("disable click? (T)"=w4133) -> ()  [unwired: 3 in, 8 out]
                      n3115 = global write "EV05全局变量1.vi" "读取超时"(w4133) -> ()
                      n3116 = global write "EV05全局变量1.vi" "流控帧"(w4133) -> ()
                      n3117 = local write "消除"(w4132) -> ()
                      n3118 = local write "控制1"(w4132) -> ()
                      n3119 = global write "EV05全局变量1.vi" "流控帧 2"(w4132) -> ()
                      n3120 = local write "写?"(w4132) -> ()
                    }
                    frame #1 {
                      n3121 = Wait Until Next ms Multiple(millisecond multiple=u32 50 ("毫秒倍数")) -> ()  [unwired: 1 out]
                    }
                    frame #2 {
                      n3122 = local read "设备索引号"() -> (w4139:u16)
                      n3123 = local read "CAN卡类型"() -> (w4140:u32)
                      n3124 = Increment(x=w4143) -> (x+1=w4142:dbl)
                      n3125 = local read "CAN端口"() -> (w4138:u16)
                      n3126 = local write "命令"(w4137) -> ()
                      n3127 = local write "命令序号"(w4135) -> ()
                      n3128 = Reshape Array(w4144, w4142) -> (w4141:dbl[])
                      n3129 = stacked-sequence {
                        tunnel: w4141 -> [_ w4158]
                        tunnel: w4140 -> [w4147 w4157]
                        tunnel: w4139 -> [w4146 w4156]
                        tunnel: w4138 -> [w4145 w4155]
                        tunnel: w4137 -> [_ w4154]
                        tunnel: w4136 -> [_ w4153]
                        tunnel: w4135 -> [_ w4152]
                        frame #0 {
                          n3130 = disable-structure shown="禁用" {
                            disable-tunnel: w4147 -> [w4150 _]
                            disable-tunnel: w4146 -> [w4149 _]
                            disable-tunnel: w4145 -> [w4148 _]
                            frame Disabled {
                              n3131 = dll-call lib="PTH1|abs FBluewave New EnergySVN_WorkBMS_Monitor_Bnet01trunkBMS_Monitor_增加二维码data\nkerneldlls\nusbcan.dll" fn="VCI_ClearBuffer"("DeviceType"=w4150, "DeviceInd"=w4149, "CANInd"=w4148) -> (error out=w4151:errorcluster)  [unwired: 4 in, 4 out]
                              n3132 = call <vilib>:"Clear Errors.vi"("error in (no error)"=w4151) -> ()  [unwired: 6 in, 1 out]
                            }
                            frame Enabled {
                            }
                          }
                        }
                        frame #1 {
                          n3133 = call "多帧发送机制(EV05).vi"("can卡类型"=w4157, "设备索引号"=w4156, "CAN端口"=w4155, "命令"=w4154, "板号"=w4153, "命令序号"=w4152, "输入数据"=w4158) -> ()  [unwired: 1 in, 12 out]
                        }
                      }
                    }
                    frame #3 {
                      n3134 = while {
                        tunnel: [w4161] -> w4159
                        i -> [w4165]
                        stop <- w4162 stop-if-true
                        n3135 = local read "强制终止读写标记"() -> (w4160:bool)
                        n3136 = global read "EV05全局变量1.vi" "读取超时"() -> (w4161:bool)
                        n3137 = Greater Or Equal?(x=w4165, y=30) -> (x >= y?=w4163:bool)
                        n3138 = Wait Until Next ms Multiple(millisecond multiple=u32 100 ("毫秒倍数")) -> ()  [unwired: 1 out]
                        n3139 = Compound Arithmetic op=OR(w4160, w4161, w4163) -> (w4162:bool)
                      }
                    }
                    frame #4 {
                      n3140 = case shown="假" w4168 {
                        tunnel: w4167 -> [w4169 w4175]
                        frame False {
                          n3141 = control-ref of="结果"() -> (w4173:refnum<vi>)
                          n3142 = Concatenate Strings(w4169, "       写入失败" ("字符串")) -> (w4172:string)
                          n3143 = Build Array(w4172) -> (w4171:string[])
                          n3144 = call "表格编辑.vi"("新元素/子数组"=w4171, "活动单元格:单元格背景色"=u32 16740749, "MCListbox引用句柄"=w4173) -> ()  [unwired: 9 out]
                        }
                        frame True {
                          n3145 = case shown="\"从板号\"" w4175 {
                            frame "假", Default {
                            }
                            frame "从板号" {
                              n3146 = local read "从板号"() -> (w4176:u8)
                              n3147 = local write "当前从板板号"(w4176) -> ()
                            }
                          }
                        }
                      }
                      n3148 = call <vilib>:"Unset Busy.vi"() -> ()  [unwired: 2 in, 10 out]
                    }
                    frame #5 {
                      n3149 = Increment(x=w4179) -> (x+1=w4178:i32)
                      n3150 = Equal?(x=w4180, y=w4178) -> (x = y?=w4177:bool)
                      n3151 = case shown="真" w4177 {
                        frame False {
                        }
                        frame True {
                          n3152 = control-ref of="结果"() -> (w4184:refnum<vi>)
                          n3153 = Concatenate Strings("写入完成" ("字符串")) -> (w4183:string)
                          n3154 = Build Array(w4183) -> (w4182:string[])
                          n3155 = call "表格编辑.vi"("新元素/子数组"=w4182, "活动单元格:单元格背景色"=u32 21937, "MCListbox引用句柄"=w4184) -> ()  [unwired: 9 out]
                        }
                      }
                    }
                  }
                }
              }
            }
            n3156 = stacked-sequence {
              tunnel: w4058 -> [_]
              frame #0 {
                n3157 = call <vilib>:"Unset Busy.vi"() -> ()  [unwired: 2 in, 10 out]
                n3158 = local write "强制终止读写标记"(FALSE ("强制停止")) -> ()
              }
            }
          }
          frame "全部写入" {
            n3159 = local read "主从选择"() -> (w4191:enum32{"主板", "从板"})
            n3160 = case shown="\"主板\", 默认" w4191 {
              tunnel: [string[] ["项目信息", "一级故障阀值", "二级故障阀值", "三级故障阀值", "加热控制参数", "充电控制参数", "电池信息"] string[] ["从板信息", "一级故障阀值", "二级故障阀值", "三级故障阀值", "均衡参数"]] -> w4188
              tunnel: [0.0 ("从板号") w4320] -> w4192
              tunnel: [w4305 _] -> w4190
              tunnel: [_ w4321] -> w4189
              frame "主板", Default {
                n3161 = stacked-sequence {
                  tunnel: [_ w4319] -> w4305
                  frame #0 {
                    n3162 = control-ref of="电池信息"() -> (w4311:refnum<vi>)
                    n3163 = control-ref of="高压参数"() -> (w4310:refnum<vi>)
                    n3164 = control-ref of="一级故障"() -> (w4313:refnum<vi>)
                    n3165 = control-ref of="一级故障 2"() -> (w4315:refnum<vi>)
                    n3166 = control-ref of="一级故障 3"() -> (w4316:refnum<vi>)
                    n3167 = control-ref of="加热控制参数"() -> (w4317:refnum<vi>)
                    n3168 = control-ref of="充电控制参数"() -> (w4318:refnum<vi>)
                    n3169 = control-ref of="项目信息"() -> (w4314:refnum<vi>)
                    n3170 = control-ref of="项目信息2"() -> (w4312:refnum<vi>)
                    n3171 = local read "主板数据"() -> (w4309:T4)
                    n3172 = Bundle(cluster=w4309, "项目信息"=w4314, "一级故障 4"=w4312, "一级故障"=w4313, "一级故障 2"=w4315, "一级故障 3"=w4316, "加热控制参数"=w4317, "充电控制参数"=w4318, "高压参数"=w4310, "电池信息"=w4311) -> (w4308:T4)
                    n3173 = local write "主板数据"(w4308) -> ()
                  }
                  frame #1 {
                    n3174 = control-ref of="主板数据"() -> (w4319:refnum<vi>)
                  }
                }
              }
              frame "从板" {
                (unwired) "均衡参数"
                n3175 = stacked-sequence {
                  tunnel: [_ w4333] -> w4321
                  frame #0 {
                    n3176 = control-ref of="从板号"() -> (w4327:refnum<vi>)
                    n3177 = control-ref of="项目信息 2"() -> (w4328:refnum<vi>)
                    n3178 = control-ref of="均衡参数"() -> (w4325:refnum<vi>)
                    n3179 = control-ref of="加热控制参数"() -> (w4329:refnum<vi>)
                    n3180 = control-ref of="一级故障(从板)"() -> (w4330:refnum<vi>)
                    n3181 = control-ref of="二级故障(从板)"() -> (w4331:refnum<vi>)
                    n3182 = control-ref of="三级故障(从板)"() -> (w4332:refnum<vi>)
                    n3183 = control-ref of="电池组信息"() -> (w4326:refnum<vi>)
                    n3184 = local read "从板信息"() -> (w4324:T2)
                    n3185 = Bundle(cluster=w4324, "从板号"=w4327, "项目信息 2"=w4328, "加热控制参数"=w4329, "一级故障(从板)"=w4330, "二级故障(从板)"=w4331, "三级故障(从板)"=w4332, "电池组信息(从板)"=w4326, "均衡参数"=w4325) -> (w4323:T2)
                    n3186 = local write "从板信息"(w4323) -> ()
                  }
                  frame #1 {
                    n3187 = control-ref of="从板信息"() -> (w4333:refnum<vi>)
                  }
                }
                n3188 = local read "从板号"() -> (w4320:u8)
              }
            }
            n3189 = Array Size(array=w4188) -> (size(s)=w4187:i32)
            n3190 = while {
              tunnel: w4188 -> [w4200] mode=indexing
              tunnel: w4191 -> [w4204]
              tunnel: w4192 -> [w4207]
              tunnel: w4190 -> [w4206]
              tunnel: w4189 -> [w4205]
              tunnel: w4187 -> [w4198]
              tunnel: [w4194] -> w4186
              i -> [w4199]
              stop <- w4195 stop-if-true
              n3191 = Increment(x=w4199) -> (x+1=w4197:i32)
              n3192 = local read "从板个数"() -> (w4212:dbl)
              n3193 = local read "快换"() -> (w4203:bool)
              n3194 = Less Or Equal?(x=w4198, y=w4197) -> (x <= y?=w4194:bool)
              n3195 = call "输入数据解析.vi"("单个参数补充"=w4212, "从板号"=w4207, "主板引用"=w4206, "从板引用"=w4205, "主板选项"=w4200, "枚举"=w4204, "快换"=w4203) -> ("输出数组"=w4211:dbl[][], "数组长度"=w4210:dbl[], "循环次数"=w4202:i32, "命令"=w4209:u32, "名称"=w4201:string[], "命令序号"=w4208:u32[])  [unwired: 2 in, 1 out]
              n3196 = case shown="\"主板\", 默认" w4204 {
                tunnel: w4199 -> [w4214 w4228]
                frame "主板", Default {
                  n3197 = case shown="6" w4214 {
                    tunnel: [T8."项目信息" ("主从板") T8."一级故障阀值" ("主从板") T8."二级故障阀值" ("主从板") T8."三级故障阀值" ("主从板") T8."控制参数" ("主从板") T8."电池信息" ("主从板")] -> w4213
                    frame 0, Default {
                      n3198 = local write "1"(TRUE ("1")) -> ()
                    }
                    frame 1 {
                      n3199 = local write "1 2"(TRUE ("1 2")) -> ()
                    }
                    frame 2 {
                      n3200 = local write "1 3"(TRUE ("1 3")) -> ()
                    }
                    frame 3 {
                      n3201 = local write "1 4"(TRUE ("1 4")) -> ()
                    }
                    frame 4, 5 {
                      n3202 = local write "1 5"(TRUE ("1 5")) -> ()
                    }
                    frame 6 {
                      n3203 = local write "1 11"(TRUE ("1 11")) -> ()
                    }
                  }
                  n3204 = local write "主板2"(w4213) -> ()
                }
                frame "从板" {
                  n3205 = case shown="1" w4228 {
                    tunnel: [T19."从板信息" ("等级 2") T19."从板信息" ("等级 2") T19."一级故障阀值" ("等级 2") T19."二级故障阀值" ("等级 2") T19."三级故障阀值" ("等级 2") T19."快换参数" ("等级 2") T14."均衡参数" ("等级 2")] -> w4227
                    frame 99, Default {
                      n3206 = local write "1 6"(TRUE ("1 6")) -> ()
                    }
                    frame 0 {
                      n3207 = local write "1 6"(TRUE ("1 6")) -> ()
                    }
                    frame 1 {
                      n3208 = local write "1 7"(TRUE ("1 7")) -> ()
                    }
                    frame 2 {
                      n3209 = local write "1 8"(TRUE ("1 8")) -> ()
                    }
                    frame 3 {
                      n3210 = local write "1 9"(TRUE ("1 9")) -> ()
                    }
                    frame 4 {
                      n3211 = local write "1 10"(TRUE ("1 10")) -> ()
                    }
                    frame 5 {
                      n3212 = local write "1 12"(TRUE ("1 10")) -> ()
                    }
                  }
                  n3213 = local write "等级 2"(w4227) -> ()
                }
              }
              n3214 = for {
                N: w4202 -> [w4245]
                tunnel: w4211 -> [w4255]
                tunnel: w4210 -> [w4254]
                tunnel: w4209 -> [w4253]
                tunnel: w4208 -> [w4251]
                tunnel: w4207 -> [w4252]
                tunnel: w4201 -> [w4248]
                tunnel: w4194 -> [w4243]
                i -> [w4244]
                n3215 = Index Array(array=w4255, index (row)=w4244) -> (element=w4250:dbl[])  [unwired: 1 in]
